vi "setUp.vi"(8 "error in (no error)":errorcluster, 11 "TestConfigurationFileBinding In":refnum<class "TestStreamToDiskTransport.lvclass">) -> (0 "error out":errorcluster, 3 "TestConfigurationFileBinding Out":refnum<class "TestStreamToDiskTransport.lvclass">)   [LabVIEW 2017, in "TestStreamToDiskTransport.lvclass"]
doc: "setUp runs prior to the test method during test execution. Use this method to initialize any object data required by your tests."
uses:
  TestStreamToDiskTransport.lvclass
  C:/Program Files (x86)/National Instruments/LabVIEW 2017/vi.lib/addons/_JKI Toolkits/VI Tester/TestCase.llb/TestCase.lvclass
  <vilib>/Utility/sysdir.llb/System Directory Type.ctl
  TestStreamToDiskTransport.lvclass/TestStreamToDiskTransport.ctl
  <vilib>/addons/_JKI Toolkits/VI Tester/TestCase.llb/TestCase.lvclass
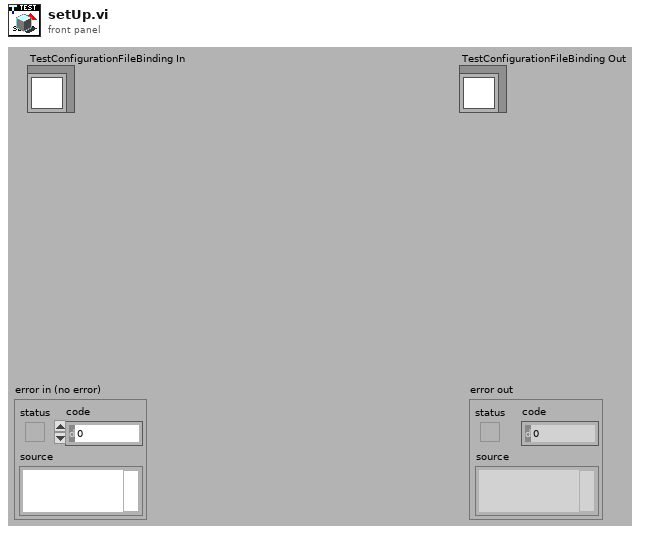
[diagram p1: front panel]
types:
  T1 = typedef "System Directory Type.ctl" = i32
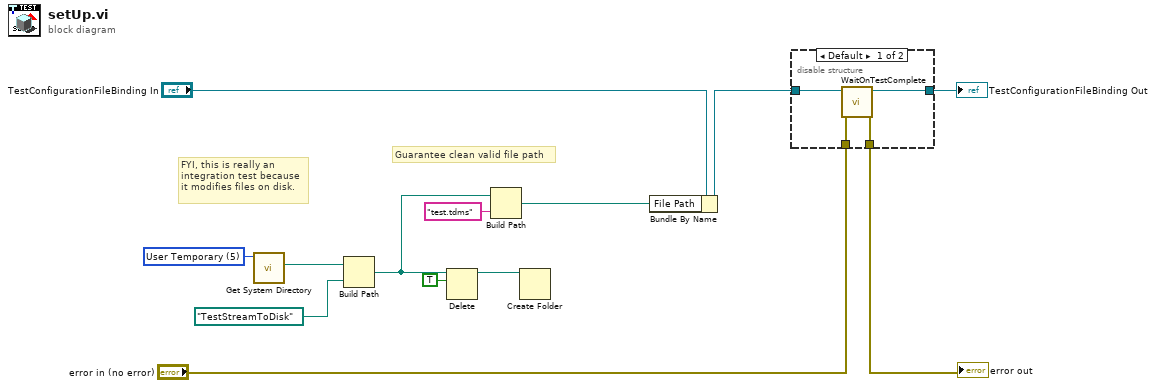
[diagram p0: block diagram]
diagram:
  w8 = T1 5 items=["User Home"=0, "User Desktop"=1, "User Documents"=2, "User Application Data"=3, "User Preferences"=4, "User Temporary"=5, "Public Documents"=6, "Public Application Data"=7, "Public Preferences"=8, "Public Cache"=13, "System Core Libraries"=9, "System Installed Libraries"=10, "Application Files"=11, "Boot Volume Root"=12] ("system directory type")
  # "Guarantee clean valid file path"
  # "FYI, this is really an\nintegration test because\nit modifies files on disk."
  n1 = call <vilib>:"Get System Directory.vi"("system directory type"=w8) -> ("system directory"=w7:path)  [unwired: 10 in]
  n2 = Build Path(base path=w7, name or relative path=path "TestStreamToDisk") -> (appended path=w3:path)
  n3 = Delete(path (use dialog)=w3, entire hierarchy (F)=TRUE) -> (deleted path=w5:path)  [unwired: 3 in, 2 out]
  n4 = Build Path(base path=w3, name or relative path="test.tdms") -> (appended path=w1:path)
  n5 = Create Folder(path (use dialog)=w5) -> ()  [unwired: 2 in, 3 out]
  n6 = Bundle By Name(cluster="TestConfigurationFileBinding In", "File Path"=w1) -> (w9:refnum<class "TestStreamToDiskTransport.lvclass">)
  n7 = disable-structure shown="Default" {
    disable-tunnel: "error in (no error)" -> [w17 w18]
    disable-tunnel: [w16 w18] -> w12
    disable-tunnel: [w15 w19] -> w10
    disable-tunnel: w9 -> [w14 w19]
    frame condition #0 (active) {
      n8 = call <vilib>:"WaitOnTestComplete.vi"("error in (no error)"=w17, "TestCase in"=w14) -> ("error out"=w16:errorcluster, "TestCase out"=w15:refnum<class "TestStreamToDiskTransport.lvclass">)  [unwired: 8 in]
    }
    frame condition #1 {
    }
  }
  "error out" <- w12
  "TestConfigurationFileBinding Out" <- w10
